vi "RegisterAppAsService.vi"(6 "service description":string, 8 "error in (no error)":errorcluster, 9 "SrvAny.exe Path":path, 10 "app path":path, 11 "service name":string) -> (0 "error out":errorcluster)   [LabVIEW 2022 SP3]
doc: "Registers an exe as a startup service for Windows."
uses:
  <vilib>/registry/registry.llb/Registry RtKey.ctl
  <vilib>/registry/registry.llb/Write Registry Value Simple STR.vi
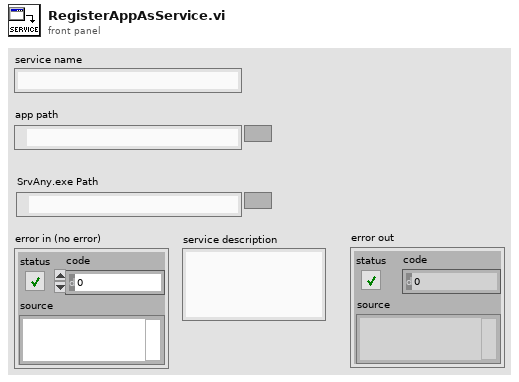
[diagram p1: front panel]
types:
  T1 = typedef "Registry RtKey.ctl" = enum32{"HKEY_CLASSES_ROOT", "HKEY_CURRENT_USER", "HKEY_LOCAL_MACHINE", "HKEY_USERS", "HKEY_PERFORMANCE_DATA", "HKEY_CURRENT_CONFIG", "HKEY_DYN_DATA"}
  T2 = typedef "Registry refnum.ctl" = refnum<k1>
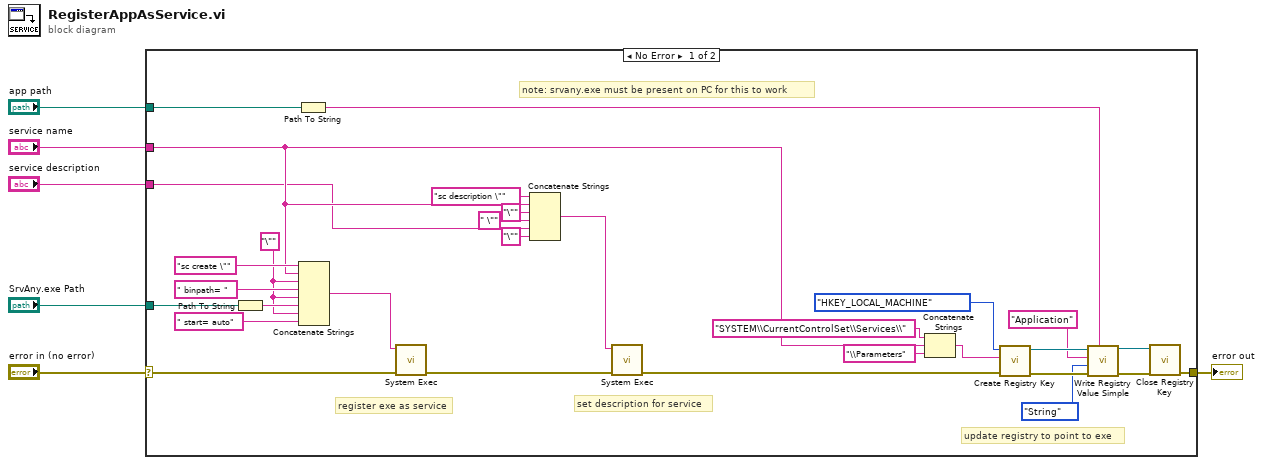
[diagram p0: block diagram]
diagram:
  n1 = case shown="No Error" "error in (no error)" {
    selector: "error in (no error)" -> [w7 w37]
    tunnel: "app path" -> [w36 _]
    tunnel: "SrvAny.exe Path" -> [w34 _]
    tunnel: "service name" -> [w17 _]
    tunnel: "service description" -> [w14 _]
    tunnel: [w8 w37] -> w2
    frame No Error {
      w31 = "\""
      # "note: srvany.exe must be present on PC for this to work"
      # "update registry to point to exe"
      # "set description for service"
      # "register exe as service"
      n2 = Path To String(path=w34) -> (string=w32:string)
      n3 = Path To String(path=w36) -> (string=w20:string)
      n4 = Concatenate Strings("sc create \"" ("string"), w17, w31, " binpath= " ("string"), w31, w32, w31, " start= auto" ("string")) -> (w12:string)
      n5 = call <vilib>:"System Exec.vi"("error in (no error)"=w7, "command line"=w12) -> ("error out"=w11:errorcluster)  [unwired: 6 in, 3 out]
      n6 = Concatenate Strings("sc description \"" ("string"), w17, "\"" ("string"), " \"" ("string"), w14, "\"" ("string")) -> (w10:string)
      n7 = call <vilib>:"System Exec.vi"("error in (no error)"=w11, "command line"=w10) -> ("error out"=w9:errorcluster)  [unwired: 6 in, 3 out]
      n8 = Concatenate Strings("SYSTEM\\CurrentControlSet\\Services\\" ("subkey"), w17, "\\Parameters" ("string")) -> (w27:string)
      n9 = call <vilib>:"Create Registry Key.vi"("error in (no error)"=w9, "subkey"=w27, "root key (HKEY_LOCAL_MACHINE)"=Registry_RtKey."HKEY_LOCAL_MACHINE") -> ("error out"=w26:errorcluster, "refnum out"=w25:T2)  [unwired: 6 in, 1 out]
      n10 = call-poly <vilib>:"Write Registry Value Simple.vi"("String/Binary data"=w20, "error in (no error)"=w26, "simple data type"=enum16{"String", "Binary", "DWORD"}."String", "value"="Application", "refnum"=w25) -> ("error out"=w22:errorcluster, "refnum out"=w21:T2)  [unwired: 3 in]
      n11 = call <vilib>:"Close Registry Key.vi"("error in (no error)"=w22, "refnum"=w21) -> ("error out"=w8:errorcluster)  [unwired: 5 in]
    }
    frame Error {
    }
  }
  "error out" <- w2
